vi "JKISM++ Compact Multiple States.vi"(9 "States in Lines":string[](array[string])) -> (2 "States":string)   [LabVIEW 2014, in "JKI-State-Machine-Plus.lvlib"]
uses:
  JKI-State-Machine-Plus.lvlib
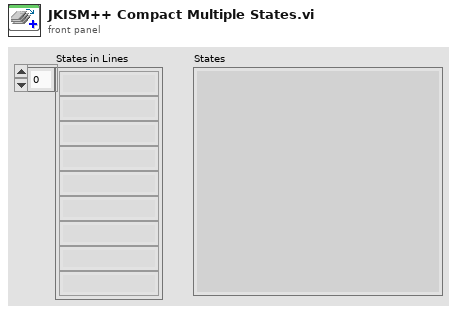
[diagram p1: front panel]
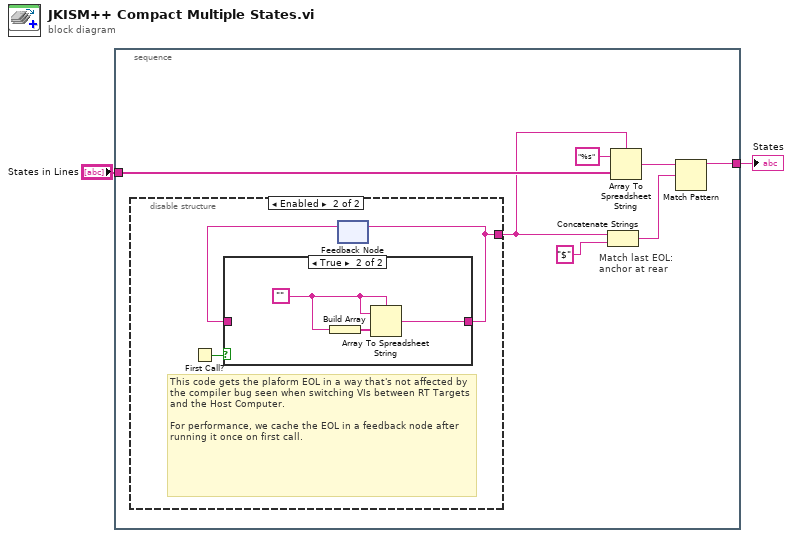
[diagram p0: block diagram]
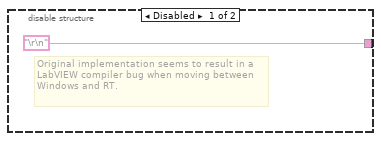
[diagram p2: hidden frame]
diagram:
  n1 = stacked-sequence {
    tunnel: [w4] -> w2
    tunnel: "States in Lines" -> [w5]
    frame #0 {
      # "Match last EOL:\nanchor at rear"
      n2 = disable-structure shown="Enabled" {
        disable-tunnel: ["\r\n" w13] -> w3
        frame Disabled {
          # "Original implementation seems to result in a LabVIEW compiler bug when moving between Windows and RT."
        }
        frame Enabled {
          # "This code gets the plaform EOL in a way that's not affected by the compiler bug seen when switching VIs between RT Targets and the Host Computer.\n\nFor performance, we cache the EOL in a feedback node after running it once on first call."
          n3 = First Call?() -> (First Call?: T/F=w12:bool)
          n4 = feedback #1() -> (w11:string)  [unwired: 1 in]
          n5 = case shown="True" w12 {
            tunnel: [w14 w15] -> w13
            tunnel: w11 -> [w14 _]
            frame False {
            }
            frame True {
              w16 = "" ("Empty String\n(hidden on FP)")
              n6 = Build Array(w16) -> (w17:string[])
              n7 = Array To Spreadsheet String(delimiter (Tab)=w16, array=w17, 3:w16) -> (spreadsheet string=w15:string)
            }
          }
          n8 = feedback-in #1(w13) -> ()
        }
      }
      n9 = Concatenate Strings(w3, "$" ("Substring")) -> (w8:string)
      n10 = Array To Spreadsheet String(delimiter (Tab)=w3, array=w5, 3:"%s" ("format string")) -> (spreadsheet string=w9:string)
      n11 = Match Pattern(string=w9, regular expression=w8) -> (before substring=w4:string)  [unwired: 1 in, 3 out]
    }
  }
  "States" <- w2
